vi "Default Instrument Setup.vi"(8 "error in (no error)":errorcluster, 11 "VISA resource name":refnum<visa-resource-name>) -> (0 "error out":errorcluster, 3 "VISA resource name out":refnum<visa-resource-name>)   [LabVIEW 2025]
doc: "Sends a default command string to the instrument whenever a new VISA session is opened, or the instrument is reset. Use this VI as a subVI for the <b>Initialize</b> and <b>Reset</b> VIs. Altering this VI could cause these two VIs to operate incorrectly."
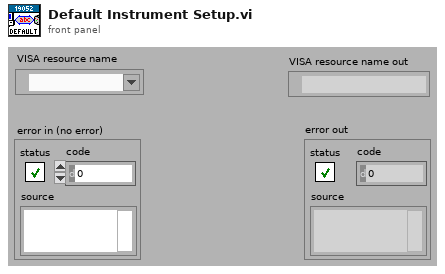
[diagram p1: front panel]
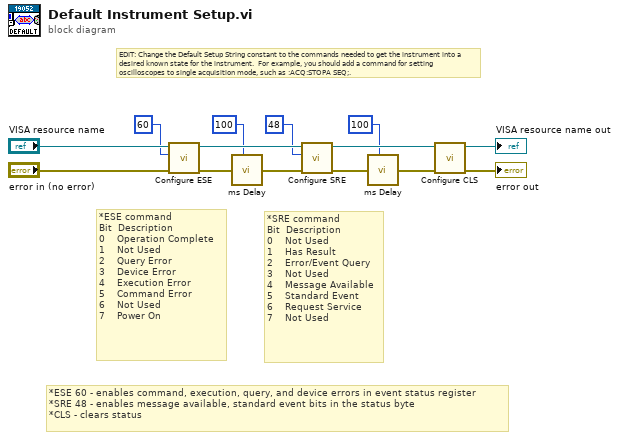
[diagram p0: block diagram]
diagram:
  # "*SRE command\nBit  Description\n0    Not Used\n1    Has Result\n2    Error/Event Query\n3    Not Used\n4    Message Available\n5    Standard Event\n6    Request Service\n7    Not Used"
  # "*ESE command\nBit  Description\n0    Operation Complete\n1    Not Used\n2    Query Error\n3    Device Error\n4    Execution Error\n5    Command Error\n6    Not Used\n7    Power On"
  # "*ESE 60 - enables command, execution, query, and device errors in event status register\n*SRE 48 - enables message available, standard event bits in the status byte\n*CLS - clears status"
  # "EDIT: Change the Default Setup String constant to the commands needed to get the instrument into a desired known state for the instrument.  For example, you should add a command for setting oscilloscopes to single acquisition mode, such as :ACQ:STOPA SEQ;."
  n1 = call "Configure ESE.vi"("error in (no error)"="error in (no error)", "decimal"=i16 60, "VISA resource name"="VISA resource name") -> ("error out"=w9:errorcluster, "VISA resource name out"=w8:refnum<visa-resource-name>)  [unwired: 7 in]
  n2 = call "ms Delay.vi"("miliseconds to wait"=u32 100 ("milliseconds to wait"), "error in (no error)"=w9) -> ("error out"=w7:errorcluster)  [unwired: 6 in, 1 out]
  n3 = call "Configure SRE.vi"("error in (no error)"=w7, "value"=u32 48, "VISA resource name"=w8) -> ("error out"=w3:errorcluster, "VISA resource name out"=w14:refnum<visa-resource-name>)  [unwired: 7 in]
  n4 = call "ms Delay.vi"("miliseconds to wait"=u32 100 ("milliseconds to wait"), "error in (no error)"=w3) -> ("error out"=w4:errorcluster)  [unwired: 6 in, 1 out]
  n5 = call "Configure CLS.vi"("error in (no error)"=w4, "VISA resource name"=w14) -> ("error out"=→"error out":errorcluster, "VISA resource name out"=→"VISA resource name out":refnum<visa-resource-name>)  [unwired: 8 in]
